vi "Close.vi"(0 "NICal5501 in":refnum<class "Cal Standard.lvclass">, 11 "error in (no error)":errorcluster) -> (4 "NICal5501 out":refnum<class "Cal Standard.lvclass">, 15 "error out":errorcluster)   [LabVIEW 2023, in "NI Cal-5501 Cal Standard.lvlib" / "Cal Standard.lvclass"]
uses:
  Cal Standard.lvclass
  Cal Standard.lvclass/Cal Standard.ctl
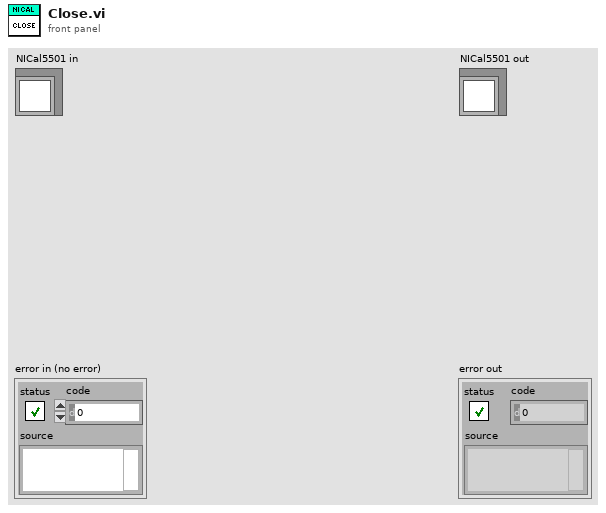
[diagram p1: front panel]
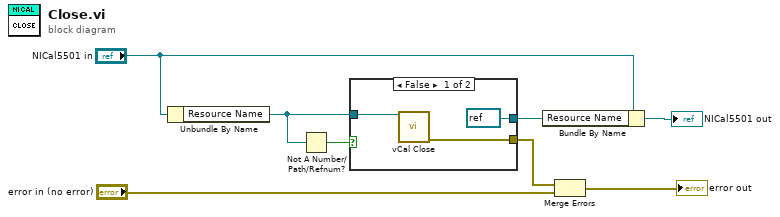
[diagram p0: block diagram]
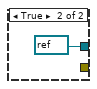
[diagram p2: hidden frame]
diagram:
  n1 = Unbundle By Name("NICal5501 in") -> ("Resource Name"=w6:refnum<k15>)
  n2 = Not A Number/Path/Refnum?(number/path/refnum=w6) -> (NaN/Path/Refnum?=w8:bool)
  n3 = case shown="False" w8 {
    tunnel: w6 -> [w11 _]
    tunnel: [w10 _] -> w7
    tunnel: [refnum<k15> refnum ("Resource Name") refnum<k15> refnum ("Resource Name")] -> w1
    frame False {
      n4 = call <instrlib>:"vCal Close.vi"("instrument handle"=w11) -> ("error out"=w10:errorcluster)  [unwired: 14 in]
    }
    frame True {
    }
  }
  n5 = Bundle By Name(cluster="NICal5501 in", "Resource Name"=w1) -> (→"NICal5501 out":refnum<class "Cal Standard.lvclass">)
  n6 = Merge Errors(w7, "error in (no error)") -> (→"error out":errorcluster)
